vi "Constants.vi"   [LabVIEW 2017, in "UDP Transceiver.lvlib" / "UDP Transceiver.lvclass"]
uses:
  UDP Transceiver.lvclass
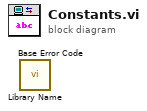
[diagram p0: block diagram]
diagram:
  n1 = call "Library Name.vi"() -> ()  [unwired: 11 in, 1 out]
  n2 = call "Base Error Code.vi"() -> ()  [unwired: 11 in, 1 out]
